vi "DeleteFinalZeros.vi"(3 "in MacroTime":u32[](array[numeric]), 4 "in MicroTime":u32[](array[numeric]), 5 "in channel":u32[](array[numeric])) -> (0 "out MacroTime":u32[](array[numeric]), 1 "out MicroTime":u32[](array[numeric]), 2 "out channel":u32[](array[numeric]))   [LabVIEW 2009]
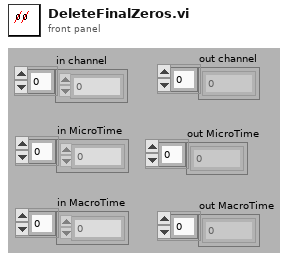
[diagram p1: front panel]
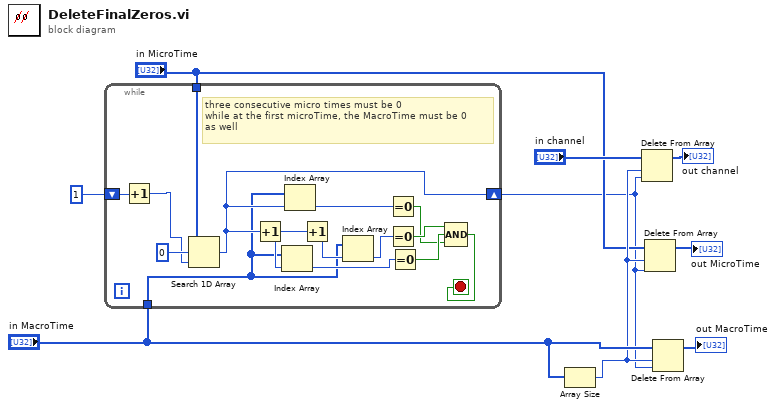
[diagram p0: block diagram]
diagram:
  n1 = while {
    tunnel: "in MacroTime" -> [w10]
    tunnel: "in MicroTime" -> [w14]
    shift-right: [w13] -> w1
    shift-left: 1 -> [w23]
    stop <- w15 stop-if-true
    # "three consecutive micro times must be 0\nwhile at the first microTime, the MacroTime must be 0\nas well"
    n2 = Increment(x=w23) -> (x+1=w22:i32)
    n3 = Search 1D Array(1D array=w14, element=u32 0 ("Element"), start index (0)=w22) -> (index of element=w13:i32)
    n4 = Increment(x=w13) -> (x+1=w20:i32)
    n5 = Index Array(array=w10, index=w20) -> (element=w19:u32)
    n6 = Index Array(array=w10, index=w13) -> (element=w12:u32)
    n7 = Increment(x=w20) -> (x+1=w21:i32)
    n8 = Index Array(array=w10, index=w21) -> (element=w18:u32)
    n9 = Equal To 0?(x=w12) -> (x = 0?=w11:bool)
    n10 = Equal To 0?(x=w18) -> (x = 0?=w17:bool)
    n11 = Equal To 0?(x=w19) -> (x = 0?=w16:bool)
    n12 = Compound Arithmetic op=AND(w17, w16, w11) -> (w15:bool)
  }
  n13 = Array Size(array="in MacroTime") -> (size(s)=w4:i32)
  n14 = Delete From Array(array="in channel", length=w4, index=w1) -> (array with subset deleted=→"out channel":u32[])  [unwired: 1 out]
  n15 = Delete From Array(array="in MicroTime", length=w4, index=w1) -> (array with subset deleted=→"out MicroTime":u32[])  [unwired: 1 out]
  n16 = Delete From Array(array="in MacroTime", length=w4, index=w1) -> (array with subset deleted=→"out MacroTime":u32[])  [unwired: 1 out]
